vi "Coordinates to Row Index.vi"(7 "Number of Initalised Rows":i32, 8 "error in (no error)":errorcluster, 10 "coords":cluster{"Horizontal":i32, "Vertical":i32}, 11 "Array ref":refnum<vi>) -> (0 "error out":errorcluster, 2 "V In Range?":bool, 3 "row index":i16)   [LabVIEW 2016]
doc: "Given a reference to a 1-D or 2-D array, and screen coordinates,\nreturn the index of the element at that location.\nTwo values are returned: col index is valid for horizontal arrays, and row index is valid for vertical arrays, both are valid for 2-D arrays"
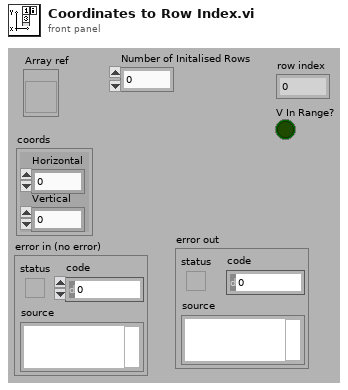
[diagram p1: front panel]
types:
  T1 = typedef "LVRectTypeDef.ctl" = cluster{"Left":i16, "Top":i16, "Right":i16, "Bottom":i16}
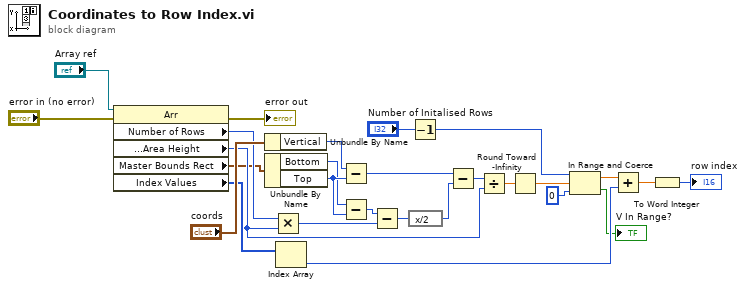
[diagram p0: block diagram]
diagram:
  n1 = property on="Property Node" class="Arr"(reference="Array ref", error in="error in (no error)") -> (error out=→"error out":errorcluster, "Number of Rows"=w5:u32, "Array Element.Bounds:Area Height"=w8:u32, "Master Bounds Rect"=w4:T1, "Index Values"=w2:u32[])  [unwired: 1 out]
  n2 = Unbundle By Name("coords") -> ("Vertical"=w22:i32)
  n3 = Unbundle By Name(w4) -> ("Bottom"=w3:i16, "Top"=w10:i16)
  n4 = Multiply(x=w5, y=w8) -> (x*y=w16:u32)
  n5 = Index Array(array=w2) -> (element=w26:u32)  [unwired: 1 in]
  n6 = Subtract(x=w22, y=w10) -> (x-y=w14:i32)
  n7 = Subtract(x=w3, y=w10) -> (x-y=w9:i16)
  n8 = Subtract(x=w9, y=w16) -> (x-y=w17:u32)
  n9 = expression code="x/2"(w17) -> (w15:u32)
  n10 = Decrement(x="Number of Initalised Rows") -> (x-1=w24:i32)
  n11 = Subtract(x=w14, y=w15) -> (x-y=w13:u32)
  n12 = Divide(x=w13, y=w8) -> (x/y=w19:dbl)
  n13 = Round Toward -Infinity(1:w19) -> (0:w12:dbl)
  n14 = In Range and Coerce(upper limit=w24, x=w12, lower limit=u32 0) -> (coerced(x)=w27:dbl, In Range?=→"V In Range?":bool)
  n15 = Add(x=w27, y=w26) -> (x+y=w25:dbl)
  n16 = To Word Integer(number=w25) -> (16bit integer=→"row index":i16)
